vi "decrement.vi"(0 "HB_Simple in":refnum<class "HB_Simple.lvclass">, 5 "error in (no error)":errorcluster) -> (14 "HB_Simple out":refnum<class "HB_Simple.lvclass">, 19 "error out":errorcluster)   [LabVIEW 2009, in "HB_BaseClass_Examples.lvlib" / "HB_Simple.lvclass"]
doc: "decrement value of x."
uses:
  HB_Simple.lvclass
  HB_Simple.lvclass/HB_Simple.ctl
  lib.lib/HGF_LVC/HGF_BaseClasses/HGF_TriggeredEvent/HGF_TriggeredEvent.lvclass
  lib.lib/HGF_LVC/HGF_BaseClasses/HGF_PVPublisher/HGF_PVPublisher.lvclass
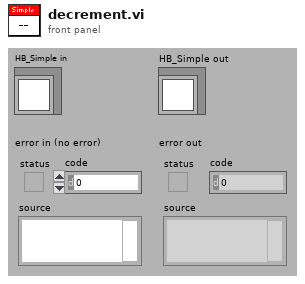
[diagram p1: front panel]
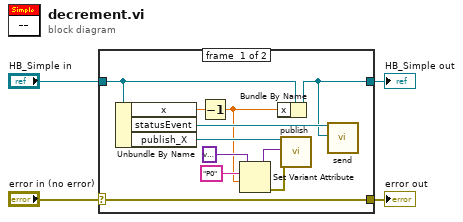
[diagram p0: block diagram]
diagram:
  n1 = case shown="No Error" "error in (no error)" {
    selector: "error in (no error)" -> [w15 w17]
    tunnel: [w15 w17] -> w3
    tunnel: [w11 w16] -> w1
    tunnel: "HB_Simple in" -> [w13 w16]
    frame #0 {
      n2 = Unbundle By Name(w13) -> ("x"=w14:dbl, "statusEvent"=w12:refnum<class "HGF_TriggeredEvent.lvclass">, "publish_X"=w6:refnum<class "HGF_PVPublisher.lvclass">)
      n3 = Decrement(x=w14) -> (x-1=w5:dbl)
      n4 = Set Variant Attribute(Variant=variant ("variant"), name="P0", value=w5) -> (Variant out=w9:variant, error out=w10:errorcluster)  [unwired: 1 in, 1 out]
      n5 = Bundle By Name(cluster=w13, "x"=w5) -> (w11:refnum<class "HB_Simple.lvclass">)
      n6 = call-dynamic "publish.vi"("HGF_PVPublisher"=w6, "data"=w9, "error in (no error)"=w10) -> ()  [unwired: 2 in, 15 out]
      n7 = call-dynamic "send.vi"("HGF_Event"=w12, "Object"=w11) -> ()  [unwired: 3 in, 15 out]
    }
    frame #1 {
    }
  }
  "error out" <- w3
  "HB_Simple out" <- w1
